vi "Lab 2 - Tank Level Control_done.vi"() -> ()   [LabVIEW 2018]
uses:
  <vilib>/DAQmx/write.llb/DAQmx Write (Analog DBL 1Chan 1Samp).vi
  Instance           3 40Saved   Lab 2 - Tank Level Control Blank .vi
  <vilib>/DAQmx/miscellaneous.llb/DAQmx Fill In Error Info.vi
panel:
  in  "Tank Control":enum16{"Tank B", "Tank A"}(ring)=enum."Tank A"
  out "Volts B":dbl
  out "Volts A":dbl
  in  "Low Level":dbl
  out "Tank Level and Limits":T1(graph)
  in  "stop":bool
  out "Time (sec)":dbl
  out "Tank B Level":dbl
  out "Tank A Level":dbl
  out "Volts to Valve":dbl
  in  "Gain":dbl
  in  "Set Value":dbl min=0.0 max=50.0
  in  "High Level":dbl
  in  "Select Controller":bool
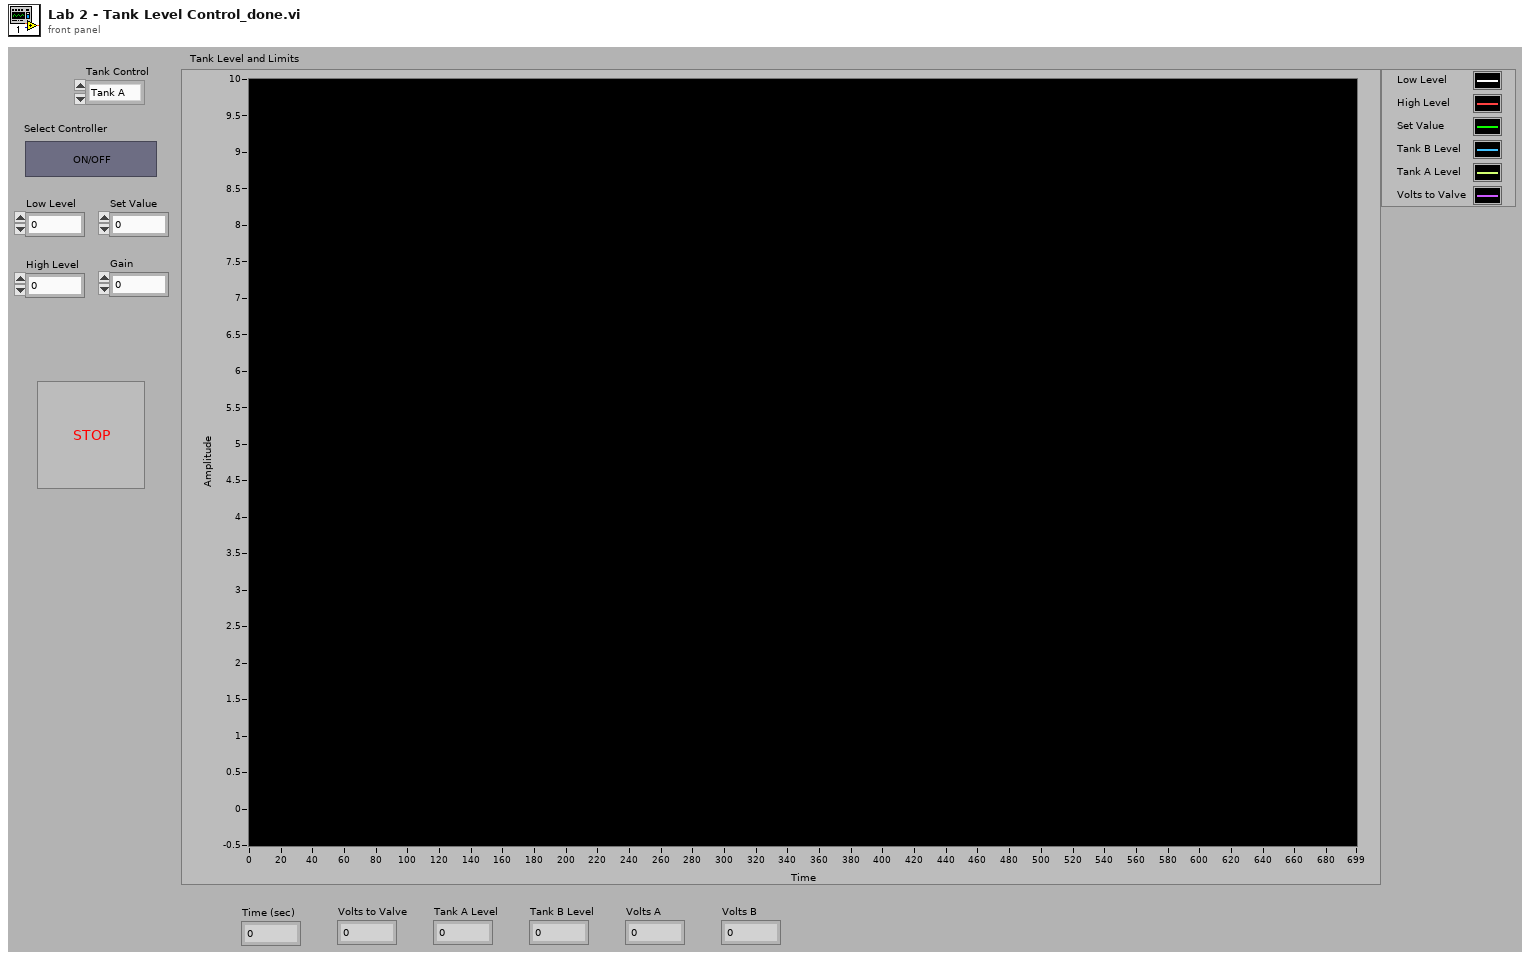
[diagram p1: front panel]
types:
  T1 = cluster{"Low Level":dbl, "High Level":dbl, "Set Value":dbl, dbl, dbl, dbl}
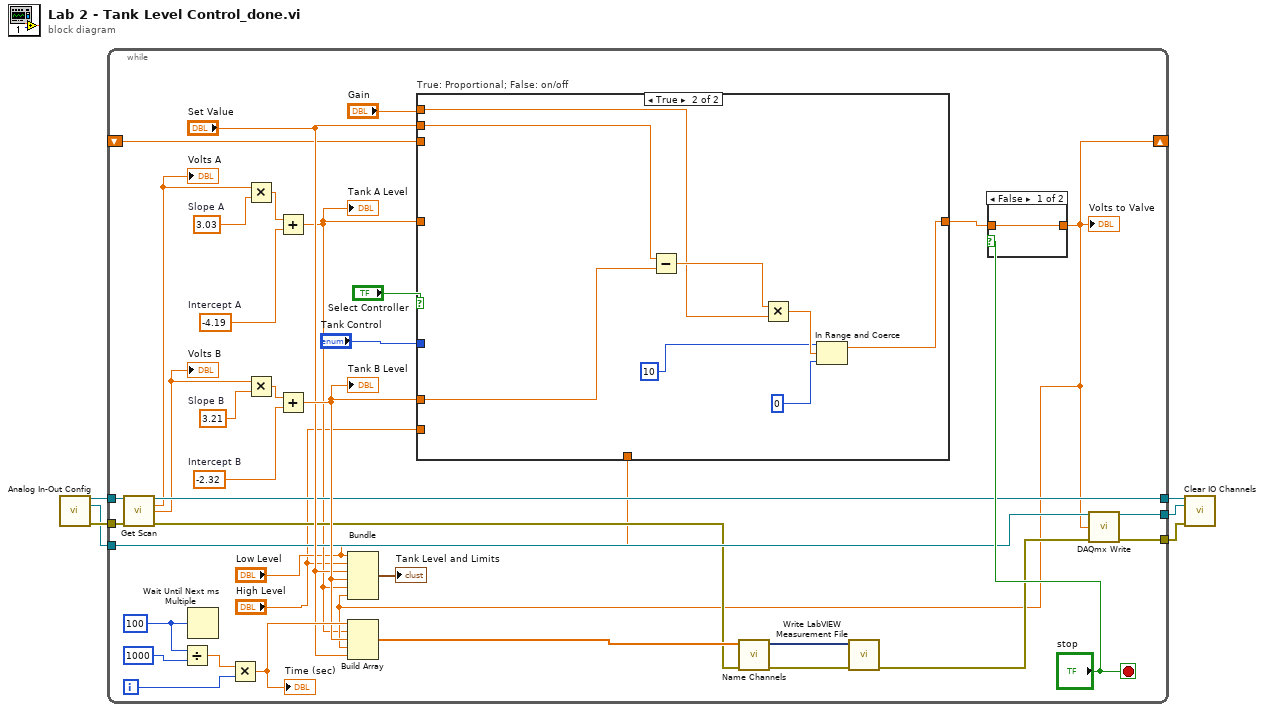
[diagram p0: block diagram]
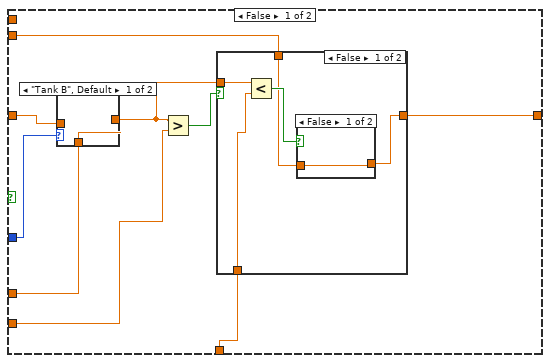
[diagram p2: hidden frame]
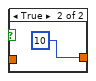
[diagram p3: hidden frame]
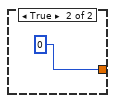
[diagram p4: hidden frame]
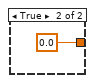
[diagram p6: hidden frame]
diagram:
  n1 = call "Analog In-Out Config.vi"() -> ("Task out A"=w6:refnum<k21>, "Task out B"=w1:refnum<k21>, "error out"=w4:errorcluster)  [unwired: 13 in]
  n2 = while {
    tunnel: w6 -> [w28]
    tunnel: w4 -> [w27]
    tunnel: [w26] -> w5
    tunnel: [w25] -> w3
    tunnel: [w24] -> w2
    tunnel: w1 -> [w23]
    shift-right: [w18] -> _
    shift-left: _ -> [w17]
    i -> [w34]
    stop <- "stop" stop-if-true
    w37 = u32 100 ("millisecond multiple")
    w13 = -4.19  # Intercept A
    w39 = -2.32  # Intercept B
    w41 = 3.21  # Slope B
    w15 = 3.03  # Slope A
    n3 = call "Get Scan.vi"("Refnum in"=w28, "error in (no error)"=w27) -> ("Refnum out"=w26:refnum<k21>, "Channel A"=w11:dbl, "Channel B"=w12:dbl, "error out"=w20:errorcluster)  [unwired: 10 in]
    "Volts A" <- w11
    "Volts B" <- w12
    n4 = Divide(x=w37, y=u32 1000) -> (x/y=w35:dbl)
    n5 = Wait Until Next ms Multiple(millisecond multiple=w37) -> ()  [unwired: 1 out]
    n6 = Multiply(x=w35, y=w34) -> (x*y=w31:dbl)
    "Time (sec)" <- w31
    n7 = Multiply(x=w11, y=w15) -> (x*y=w14:dbl)
    n8 = Multiply(x=w12, y=w41) -> (x*y=w40:dbl)
    n9 = Add(x=w14, y=w13) -> (x+y=w16:dbl)
    "Tank A Level" <- w16
    n10 = Add(x=w40, y=w39) -> (x+y=w30:dbl)
    "Tank B Level" <- w30
    n11 = case "True: Proportional; False: on/off" shown="True" "Select Controller" {
      tunnel: "Gain" -> [_ w68]
      tunnel: "Set Value" -> [_ w70]
      tunnel: w30 -> [w50 w67]
      tunnel: w17 -> [w44 _]
      tunnel: w16 -> [w51 _]
      tunnel: "Tank Control" -> [w52 _]
      tunnel: "Low Level" -> [w46 _]
      tunnel: "High Level" -> [w49 _]
      tunnel: [w45 w63] -> w7
      frame False {
        n12 = case shown="\"Tank B\", Default" w52 {
          tunnel: w51 -> [_ w62]
          tunnel: [w61 w62] -> w47
          tunnel: w50 -> [w61 _]
          frame "Tank B", Default {
          }
          frame "Tank A" {
          }
        }
        n13 = Greater?(x=w47, y=w49) -> (0:w48:bool)
        n14 = case shown="False" w48 {
          tunnel: w47 -> [w55 _]
          tunnel: w46 -> [w56 _]
          tunnel: [w54 0] -> w45
          tunnel: w44 -> [w53 _]
          frame False {
            n15 = Less?(x=w55, y=w56) -> (x < y?=w57:bool)
            n16 = case shown="False" w57 {
              tunnel: [w58 10] -> w54
              tunnel: w53 -> [w58 _]
              frame False {
              }
              frame True {
              }
            }
          }
          frame True {
          }
        }
      }
      frame True {
        n17 = Subtract(x=w70, y=w67) -> (x-y=w69:dbl)
        n18 = Multiply(x=w69, y=w68) -> (x*y=w66:dbl)
        n19 = In Range and Coerce(upper limit=10, x=w66, lower limit=0) -> (coerced(x)=w63:dbl)  [unwired: 1 out]
      }
    }
    n20 = case shown="False" "stop" {
      tunnel: [w71 0.0] -> w18
      tunnel: w7 -> [w71 _]
      frame False {
      }
      frame True {
      }
    }
    "Volts to Valve" <- w18
    n21 = Bundle("Low Level"="Low Level", "High Level"="High Level", "Set Value"="Set Value", w30, w16, w18) -> (→"Tank Level and Limits":T1)  [unwired: 1 in]
    n22 = Build Array(w31, w16, w30, w18, "Set Value") -> (w32:dbl[])
    n23 = call "Name Channels.vi"("error in (no error)"=w20, "Array"=w32) -> ("error out"=w21:errorcluster, "Dynamic Data"=w22:dynamicdata)  [unwired: 8 in]
    n24 = call "Write LabVIEW Measurement File"("error in (no error)"=w21, "Signals"=w22) -> ("error out"=w19:errorcluster)  [unwired: 7 in, 2 out]
    n25 = call-poly <vilib>:"DAQmx Write.vi"("task/channels in"=w23, "data"=w18, "error in"=w19) -> ("task out"=w25:refnum<k21>, "error out"=w24:errorcluster)  [unwired: 10 in, 1 out]
  }
  n26 = call "Clear IO Channels.vi"("Refnum in"=w5, "task out"=w3, "error in (no error)"=w2) -> ()  [unwired: 13 in]
